vi "CRYCursor Resize in Graph Window.vi"(9 "Pane Ref":refnum<vi>, 10 "input cluster":T1, 11 "Graph Cursor Ref":refnum<vi>) -> ()   [LabVIEW 2013]
uses:
  <vilib>/Utility/miscctls.llb/LVRectTypeDef.ctl
  <vilib>/Utility/miscctls.llb/LVBoundsTypeDef.ctl
  <vilib>/Utility/miscctls.llb/LVPositionTypeDef.ctl
  <vilib>/Utility/miscctls.llb/LVRowAndColumnTypeDef.ctl
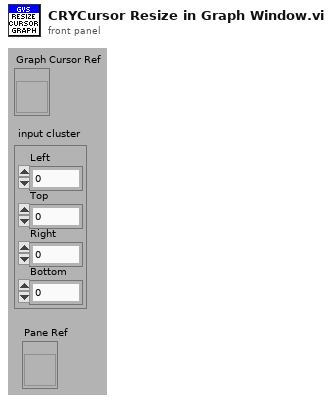
[diagram p1: front panel]
types:
  T1 = typedef "LVRectTypeDef.ctl" = cluster{"Left":i16, "Top":i16, "Right":i16, "Bottom":i16}
  T2 = typedef "LVPointTypeDef.ctl" = cluster{"Horizontal":i16, "Vertical":i16}
  T3 = typedef "LVBoundsTypeDef.ctl" = cluster{"Width":u32, "Height":u32}
  T4 = typedef "LVPositionTypeDef.ctl" = cluster{"Left":i32, "Top":i32}
  T5 = typedef "LVRowAndColumnTypeDef.ctl" = cluster{"Row":i32, "Column":i32}
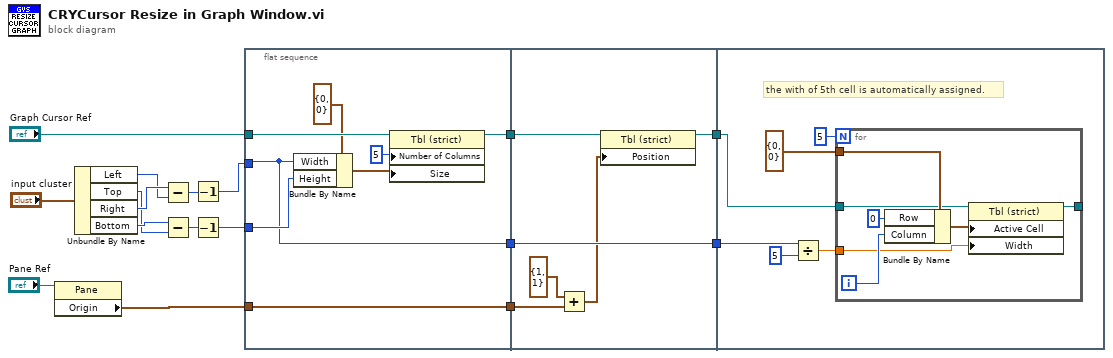
[diagram p0: block diagram]
diagram:
  n1 = property class="Pane"(reference="Pane Ref") -> ("Origin"=w6:T2)  [unwired: 1 in, 2 out]
  n2 = Unbundle By Name("input cluster") -> ("Left"=w11:i16, "Top"=w10:i16, "Right"=w17:i16, "Bottom"=w16:i16)
  n3 = Subtract(x=w17, y=w11) -> (x-y=w14:i16)
  n4 = Subtract(x=w16, y=w10) -> (x-y=w15:i16)
  n5 = Decrement(x=w14) -> (x-1=w12:i16)
  n6 = Decrement(x=w15) -> (x-1=w13:i16)
  n7 = flat-sequence {
    tunnel: w13 -> [w25]
    tunnel: w12 -> [w20]
    tunnel: w6 -> [w22]
    tunnel: "Graph Cursor Ref" -> [w23]
    tunnel: [w24] -> w4
    tunnel: [w22] -> w2
    tunnel: [w20] -> w1
    tunnel: [w31] -> w5
    tunnel: w4 -> [w30]
    tunnel: [w29] -> w3
    tunnel: w2 -> [w27]
    tunnel: w1 -> [w31]
    tunnel: w5 -> [w32]
    tunnel: w3 -> [w33]
    frame #0 {
      n8 = Bundle By Name(cluster=T3 {"Width"=0, "Height"=0} ("Size"), "Width"=w20, "Height"=w25) -> (w18:T3)
      n9 = property on="Property Node" class="Tbl (strict)"(reference=w23, "Number of Columns"=u32 5, "Size"=w18) -> (reference out=w24:refnum<vi>)  [unwired: 1 in, 1 out]
    }
    frame #1 {
      n10 = Add(x=T4 {"Left"=1, "Top"=1} ("Position"), y=w27) -> (x+y=w26:T4)
      n11 = property class="Tbl (strict)"(reference=w30, "Position"=w26) -> (reference out=w29:refnum<vi>)  [unwired: 1 in, 1 out]
    }
    frame #2 {
      # "the with of 5th cell is automatically assigned."
      n12 = Divide(x=w32, y=5) -> (x/y=w34:dbl)
      n13 = for {
        N: 5 -> [_]
        tunnel: T5 {"Row"=0, "Column"=0} ("Active Cell:Active Cell") -> [w44]
        tunnel: w34 -> [w40]
        tunnel: w33 -> [w39]
        tunnel: [w38] -> _
        i -> [w42]
        n14 = Bundle By Name(cluster=w44, "Row"=0, "Column"=w42) -> (w41:T5)
        n15 = property on="Property Node" class="Tbl (strict)"(reference=w39, "Active Cell"=w41, "Width"=w40) -> (reference out=w38:refnum<vi>)  [unwired: 1 in, 1 out]
      }
    }
  }
